vi "Write Channel's to Tree.vi"(7 "Data Cluster In":T7={"UI Reference"={"All Ctrl's Label's"=[], "ChannelListTree"=refnum, "All Object Ref"=[]}, "Tree Selection"={"Selected Channel"="", "Selected Interface"="", "Selected HW"="", "Tree Root Name"="", "Selected Module"=""}, "Selected File Path"=path "", "Selected HW"={"Slctd Hw Name"=[], "Slctd HW IP"=[]}, "Channel Config Path"=path "", "Interface Data"={"DO Channel's"=[]}, "General Info's"={"Idnentification name"=""}, "Status"="", "Channel Type's"={"Channel Type"=enum."Voltage", "Sub-Type"=enum."Pressure"}, "This VI"=refnum, "Hardware Information "=variant(variant[] [])}, 8 "error in (no error)":errorcluster, 10 "Interface Data":T1 {"AI Config Data's"."Analog Input Timing"."sample mode" items=["Finite Samples"=10178, "Continuous Samples"=10123, "Hardware Timed Single Point"=12522]}, 11 "File Name":string="File Name") -> (0 "error out":errorcluster, 5 "Data Cluster Out":T7={"UI Reference"={"All Ctrl's Label's"=[], "ChannelListTree"=refnum, "All Object Ref"=[]}, "Tree Selection"={"Selected Channel"="", "Selected Interface"="", "Selected HW"="", "Tree Root Name"="", "Selected Module"=""}, "Selected File Path"=path "", "Selected HW"={"Slctd Hw Name"=[], "Slctd HW IP"=[]}, "Channel Config Path"=path "", "Interface Data"={"DO Channel's"=[]}, "General Info's"={"Idnentification name"=""}, "Status"="", "Channel Type's"={"Channel Type"=enum."Voltage", "Sub-Type"=enum."Pressure"}, "This VI"=refnum, "Hardware Information "=variant(variant[] [])})   [LabVIEW 2021, in "Configuration.lvlib"]
uses:
  Configuration.lvlib
  Module Data--cluster.ctl
  Host-Control's/Configuration UI Reference.ctl
  DO Channel's.ctl
  Config-Channel Type.ctl
  Channel Sub-Type.ctl
  All Interface Data.ctl
  Analog Input Single Channel Data--Cluster.ctl
  Analog Output/Controls/AO Timing Cluster.ctl
  <vilib>/National Instruments/Tree Map/API/List Roots.vi
  <vilib>/National Instruments/Tree Map/Utility/Into Tree Control Items.vi
  <vilib>/National Instruments/Tree Map/Tree Map.lvlib
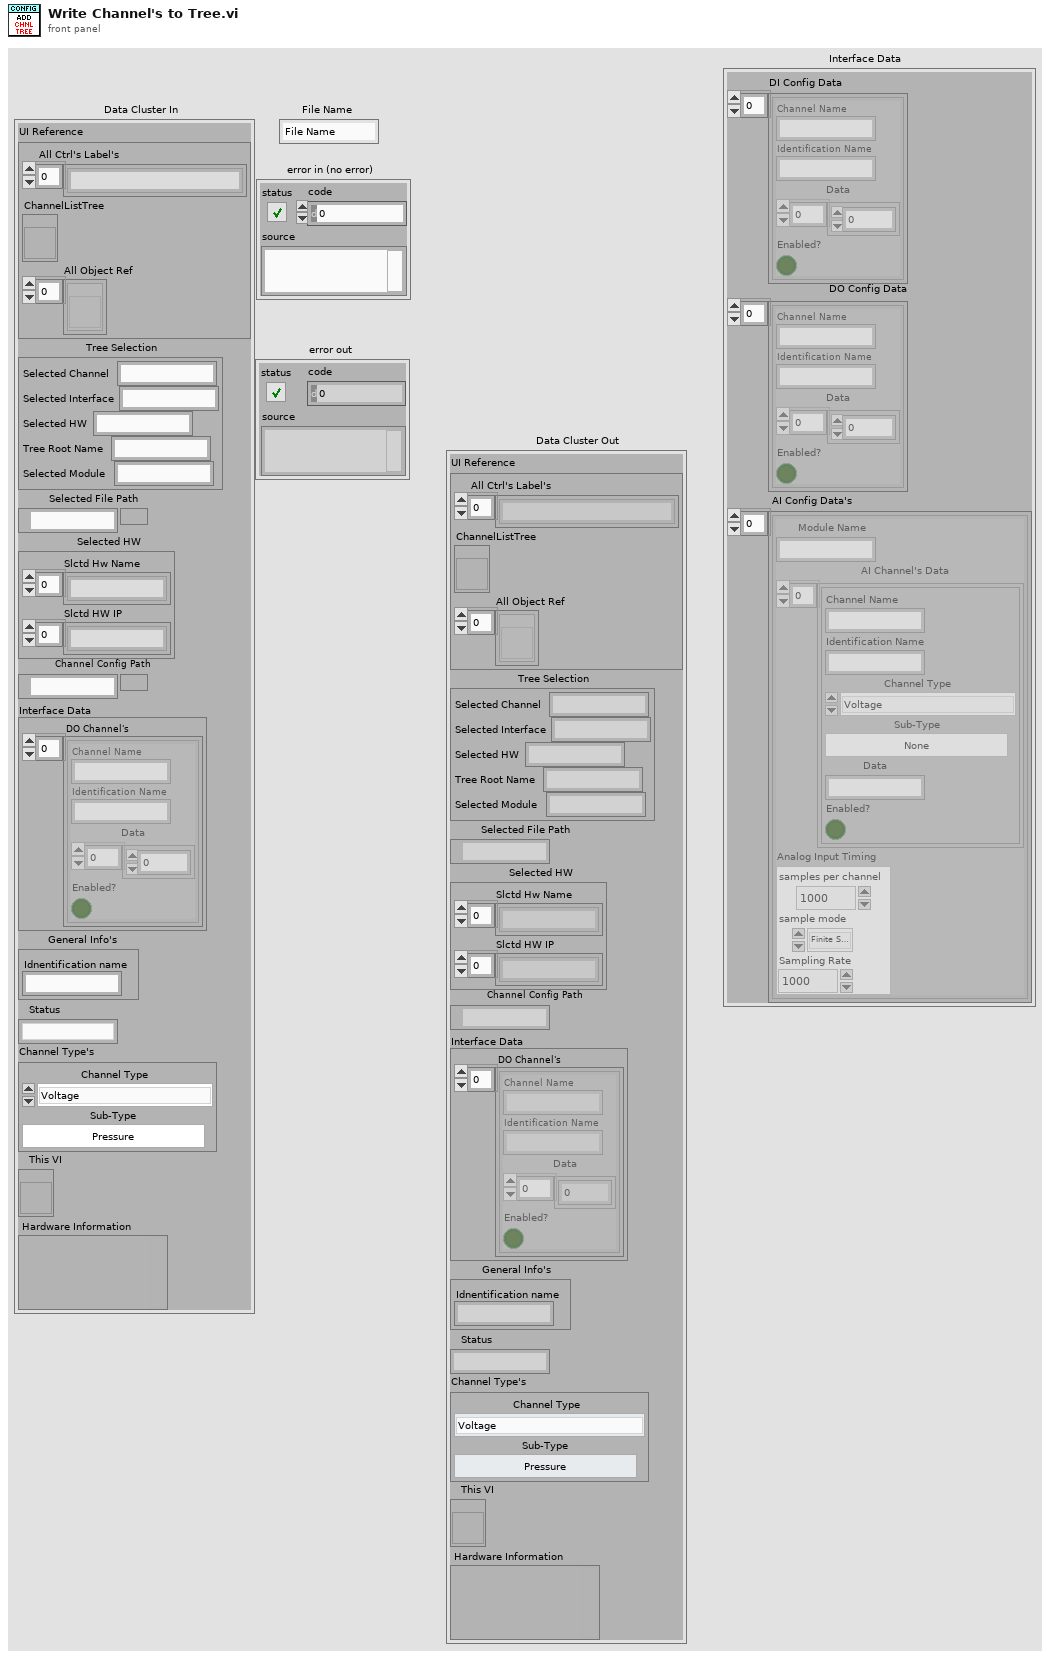
[diagram p1: front panel]
types:
  T1 = typedef "Configuration.lvlib/All Interface Data.ctl" = cluster{"DI Config Data":T2, "DO Config Data":T2, "AI Config Data's":cluster{"Module Name":string, "AI Channel's Data":T3[], "Analog Input Timing":T6}[]}
  T2 = typedef "Configuration.lvlib/DO Channel's.ctl" = cluster{"Channel Name":string, "Identification Name":string, "Data":u8[], "Enabled?":bool}[]
  T3 = typedef "Configuration.lvlib/Analog Input Single Channel Data--Cluster.ctl" = cluster{"Channel Name":string, "Identification Name":string, "Channel Type":T4, "Sub-Type":T5, "Data":string, "Enabled?":bool}
  T4 = typedef "Configuration.lvlib/Config-Channel Type.ctl" = enum16{"Voltage", "Current", "Thermocouple", "Acclerometer"}
  T5 = typedef "Configuration.lvlib/Channel Sub-Type.ctl" = enum16{"None", "Pressure", "Force"}
  T6 = typedef "AO Timing Cluster.ctl" = cluster{"samples per channel":i32, "sample mode":i32, "Sampling Rate":dbl}
  T7 = typedef "Configuration.lvlib/Module Data--cluster.ctl" = cluster{"UI Reference":T8, "Tree Selection":cluster{"Selected Channel":string, "Selected Interface":string, "Selected HW":string, "Tree Root Name":string, "Selected Module":string}, "Selected File Path":path, "Selected HW":cluster{"Slctd Hw Name":string[], "Slctd HW IP":string[]}, "Channel Config Path":path, "Interface Data":cluster{"DO Channel's":T2}, "General Info's":cluster{"Idnentification name":string}, "Status":string, "Channel Type's":cluster{"Channel Type":T4, "Sub-Type":T5}, "This VI":refnum<vi>, "Hardware Information ":variant}
  T8 = typedef "Configuration UI Reference.ctl" = cluster{"All Ctrl's Label's":string[], "ChannelListTree":refnum<vi>, "All Object Ref":refnum<vi>[]}
  T9 = cluster{"Module Name":string, "AI Channel's Data":T3[], "Analog Input Timing":T6}[]
  T10 = typedef "Tree Map.lvlib/Tree Map Data.ctl" = map{string, cluster{"Child Paths Set":set{string}, "Name":string, "Data":string, "Attributes":map{string, string}}}
  T11 = cluster{"Left Cell String":string, "Child Text":string[], "Child Tag":string, "Item Indent":i32, "Child Only?":bool, "Glyph Index":i32}[]
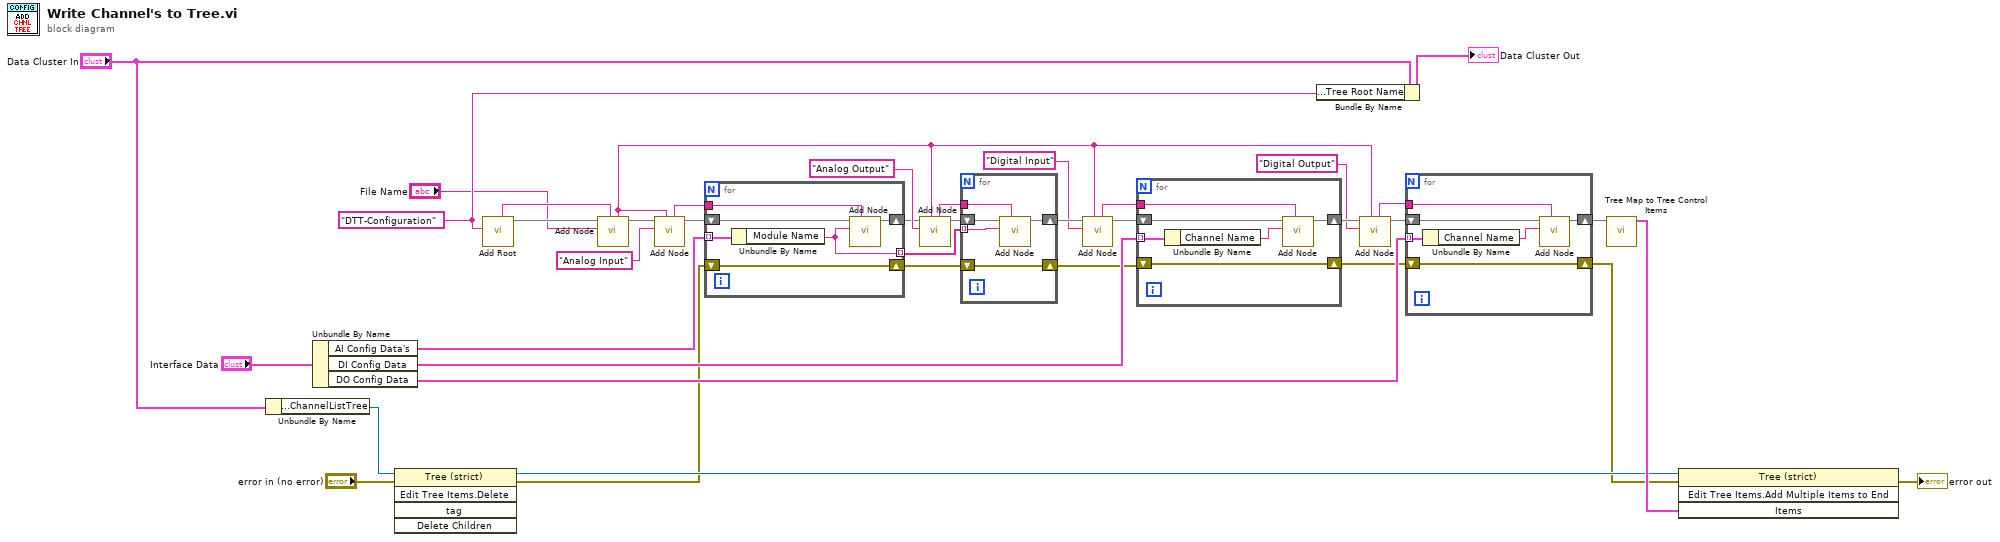
[diagram p0: block diagram]
diagram:
  w32 = "DTT-Configuration" ("New Root Name")
  n1 = Unbundle By Name("Data Cluster In") -> ("UI Reference.ChannelListTree"=w33:refnum<vi>)
  n2 = Unbundle By Name("Interface Data") -> ("AI Config Data's"=w27:T9, "DI Config Data"=w7:T2, "DO Config Data"=w6:T2)
  n3 = invoke class="Tree (strict)" method="Edit Tree Items.Delete"(reference=w33, error in="error in (no error)") -> (reference out=w34:refnum<vi>, error out=w5:errorcluster)  [unwired: 3 in, 3 out]
  n4 = call <vilib>:"Add Root.vi"("New Root Name"=w32) -> ("Tree Map Out"=w35:T10, "Root Path"=w36:string)  [unwired: 9 in]
  n5 = call <vilib>:"Add Node.vi"("Parent Path"=w36, "New Node Name"="File Name", "Tree Map In"=w35) -> ("Tree Map Out"=w22:T10, "New Node Path"=w11:string)  [unwired: 6 in, 1 out]
  n6 = call <vilib>:"Add Node.vi"("Parent Path"=w11, "New Node Name"="Analog Input", "Tree Map In"=w22) -> ("Tree Map Out"=w24:T10, "New Node Path"=w25:string)  [unwired: 6 in, 1 out]
  n7 = for {
    shift-right: [w45] -> w20
    shift-left: w24 -> [w43]
    tunnel: w25 -> [w44]
    tunnel: w27 -> [w42] mode=indexing
    tunnel: [w41] -> w9 mode=indexing
    shift-right: [w40] -> w4
    shift-left: w5 -> [w40]
    n8 = Unbundle By Name(w42) -> ("Module Name"=w41:string)
    n9 = call <vilib>:"Add Node.vi"("Parent Path"=w44, "New Node Name"=w41, "Tree Map In"=w43) -> ("Tree Map Out"=w45:T10)  [unwired: 6 in, 2 out]
  }
  n10 = call <vilib>:"Add Node.vi"("Parent Path"=w11, "New Node Name"="Analog Output", "Tree Map In"=w20) -> ("Tree Map Out"=w19:T10, "New Node Path"=w21:string)  [unwired: 6 in, 1 out]
  n11 = for {
    shift-right: [w50] -> w14
    shift-left: w19 -> [w47]
    tunnel: w9 -> [w49] mode=indexing
    tunnel: w21 -> [w48]
    shift-right: [w46] -> w2
    shift-left: w4 -> [w46]
    n12 = call <vilib>:"Add Node.vi"("Parent Path"=w48, "New Node Name"=w49, "Tree Map In"=w47) -> ("Tree Map Out"=w50:T10)  [unwired: 6 in, 2 out]
  }
  n13 = call <vilib>:"Add Node.vi"("Parent Path"=w11, "New Node Name"="Digital Input", "Tree Map In"=w14) -> ("Tree Map Out"=w18:T10, "New Node Path"=w17:string)  [unwired: 6 in, 1 out]
  n14 = for {
    shift-right: [w56] -> w12
    shift-left: w18 -> [w54]
    tunnel: w17 -> [w55]
    tunnel: w7 -> [w53] mode=indexing
    shift-right: [w51] -> w3
    shift-left: w2 -> [w51]
    n15 = Unbundle By Name(w53) -> ("Channel Name"=w52:string)
    n16 = call <vilib>:"Add Node.vi"("Parent Path"=w55, "New Node Name"=w52, "Tree Map In"=w54) -> ("Tree Map Out"=w56:T10)  [unwired: 6 in, 2 out]
  }
  n17 = Bundle By Name(cluster="Data Cluster In", "Tree Selection.Tree Root Name"=w32) -> (→"Data Cluster Out":T7)
  n18 = call <vilib>:"Add Node.vi"("Parent Path"=w11, "New Node Name"="Digital Output", "Tree Map In"=w12) -> ("Tree Map Out"=w15:T10, "New Node Path"=w16:string)  [unwired: 6 in, 1 out]
  n19 = for {
    shift-right: [w62] -> w37
    shift-left: w15 -> [w60]
    tunnel: w16 -> [w61]
    tunnel: w6 -> [w59] mode=indexing
    shift-right: [w57] -> w1
    shift-left: w3 -> [w57]
    n20 = Unbundle By Name(w59) -> ("Channel Name"=w58:string)
    n21 = call <vilib>:"Add Node.vi"("Parent Path"=w61, "New Node Name"=w58, "Tree Map In"=w60) -> ("Tree Map Out"=w62:T10)  [unwired: 6 in, 2 out]
  }
  n22 = call <vilib>:"Tree Map to Tree Control Items.vi"("Tree Map In"=w37) -> ("Tree Control Items"=w38:T11)  [unwired: 10 in]
  n23 = invoke class="Tree (strict)" method="Edit Tree Items.Add Multiple Items to End"(reference=w34, error in=w1, "Items"=w38) -> (error out=→"error out":errorcluster)  [unwired: 1 in, 3 out]
